vi "DesactivarDatosBandeja.vi"(11 "Array":refnum<vi>[](array[refnum])) -> ()   [LabVIEW 2019]
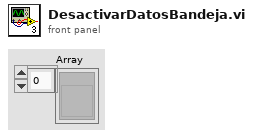
[diagram p1: front panel]
types:
  T1 = enum8{"Enabled", "Disabled", "Disabled and Grayed Out"}
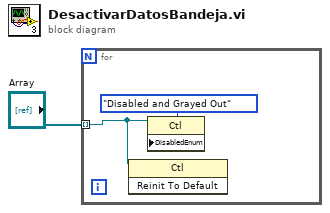
[diagram p0: block diagram]
diagram:
  n1 = for {
    tunnel: "Array" -> [w2] mode=indexing
    n2 = invoke class="Ctl" method="Reinit To Default"(reference=w2) -> ()  [unwired: 2 in, 3 out]
    n3 = property class="Ctl"(reference=w2, "DisabledEnum"=T1."Disabled and Grayed Out" ("Disabled")) -> ()  [unwired: 1 in, 2 out]
  }
